vi "Get Configured Monitoring Channels.vi"(8 "error in (no error)":errorcluster, 11 "VeriStand Data Sharing Framework in":refnum<class "VeriStand DSF.lvclass">) -> (0 "error out":errorcluster, 1 "monitoring channels refs":T1[](array[typedef]) format="%.0x", 2 "monitoring channel offsets":u64[](array[numeric]) format="%.0x", 3 "VeriStand Data Sharing Framework out":refnum<class "VeriStand DSF.lvclass">)   [LabVIEW 2017, in "DSF Engine.lvlib" / "VeriStand DSF.lvclass"]
uses:
  VeriStand DSF.lvclass
  <vilib>/NI Veristand/Custom Device API/Custom Device Item Ref.ctl
  VeriStand DSF.lvclass/VeriStand DSF.ctl
  <vilib>/NI Veristand/Custom Device API/Data Access Type.ctl
  <vilib>/NI Veristand/Custom Device API/Custom Device API.lvlib
  Shared/DSF Shared.lvlib
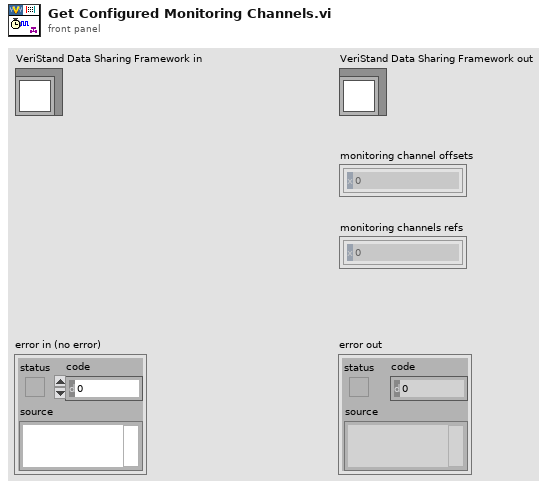
[diagram p1: front panel]
types:
  T1 = typedef "Custom Device API.lvlib/Custom Device Item Ref.ctl" = u64
  T2 = typedef "Custom Device API.lvlib/Data Access Type.ctl" = enum16{"Read", "Write"}
  T3 = typedef "Custom Device API.lvlib/Data Reference.ctl" = i32
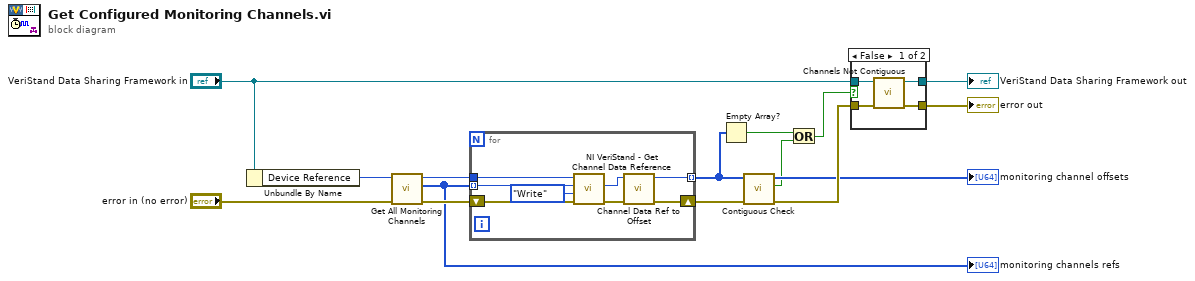
[diagram p0: block diagram]
diagram:
  n1 = Unbundle By Name("VeriStand Data Sharing Framework in") -> ("Device Reference"=w6:T1)
  n2 = call "Get All Monitoring Channels.vi"("error in (no error)"="error in (no error)", "Item Ref in"=w6) -> ("error out"=w14:errorcluster, "performance channels refs"=w7:T1[], "Item Ref out"=w5:T1)  [unwired: 7 in]
  "monitoring channels refs" <- w7
  n3 = for {
    shift-right: [w22] -> w13
    shift-left: w14 -> [w21]
    tunnel: [w19] -> w4 mode=indexing
    tunnel: w5 -> [w17]
    tunnel: w7 -> [w16] mode=indexing
    n4 = call <vilib>:"NI VeriStand - Get Channel Data Reference.vi"("error in (no error)"=w21, "Access"=Data_Access_Type."Write", "Channel Ref in"=w16, "Device Ref in"=w17) -> ("error out"=w23:errorcluster, "Channel Data Reference"=w20:T3)  [unwired: 5 in, 1 out]
    n5 = call "Channel Data Ref to Offset.vi"("error in (no error)"=w23, "Channel Data Reference"=w20) -> ("error out"=w22:errorcluster, "channel offset"=w19:u64)  [unwired: 8 in]
  }
  n6 = Empty Array?(array=w4) -> (empty?=w3:bool)
  n7 = call "Contiguous Check.vi"("error in (no error)"=w13, "channel offsets in"=w4) -> ("error out"=w9:errorcluster, "contiguous?"=w2:bool, "channel offsets out"=→"monitoring channel offsets":u64[])  [unwired: 7 in]
  n8 = Or(x=w3, y=w2) -> (x .or. y?=w1:bool)
  n9 = case shown="False" w1 {
    tunnel: "VeriStand Data Sharing Framework in" -> [w27 w29]
    tunnel: [w26 w29] -> w11
    tunnel: [w25 w28] -> w10
    tunnel: w9 -> [w24 w28]
    frame False {
      n10 = call "Channels Not Contiguous.vi"("error in (no error)"=w24, "VeriStand DSF in"=w27) -> ("error out"=w25:errorcluster, "VeriStand DSF out"=w26:refnum<class "VeriStand DSF.lvclass">)  [unwired: 8 in]
    }
    frame True {
    }
  }
  "error out" <- w10
  "VeriStand Data Sharing Framework out" <- w11
